vi "DetectionObjectiveStand_Analog.vi"(4 "stand Z vol Backward samp info":cluster{"Fs":dbl, "#s":dbl}={"Fs"=500000.0, "#s"=68421.0}, 6 "stand Z vol Acquisition samp info":cluster{"Fs":dbl, "#s":dbl}={"Fs"=500000.0, "#s"=131579.0}, 7 "Objective scan volt":dbl=5.0, 8 "error in (no error)":errorcluster, 9 "stand Z vol Backward time (s)":dbl=0.13684210526315793, 10 "stand Z vol Acquisition time (s)":dbl=0.2631578947368421, 11 "Steps per volume":dbl=25.0) -> (0 "error out":errorcluster, 3 "DetectionObjectiveStand":waveform(dbl))   [LabVIEW 2018]
panel:
  out "Preview":waveform(dbl)(graph)
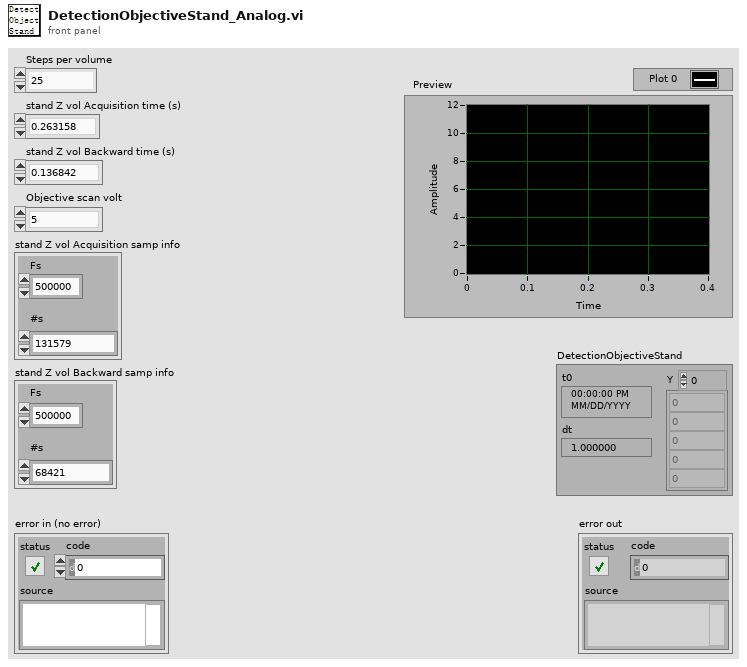
[diagram p1: front panel]
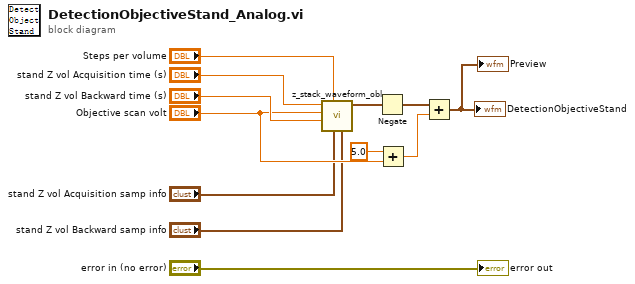
[diagram p0: block diagram]
diagram:
  n1 = call "z_stack_waveform_obl.vi"("Z stack backward"="stand Z vol Backward samp info", "Z stack acquisition"="stand Z vol Acquisition samp info", "Steps per Volume"="Steps per volume", "Backward Time (s)"="stand Z vol Backward time (s)", "SPECIFIC scan volt"="Objective scan volt", "Aquisition Time (s)"="stand Z vol Acquisition time (s)") -> ("WaveformOut"=w9:waveform(dbl))  [unwired: 5 in]
  n2 = Negate(x=w9) -> (-x=w12:waveform(dbl))
  n3 = Add(x=5.0, y="Objective scan volt") -> (x+y=w10:dbl)
  n4 = Add(x=w12, y=w10) -> (x+y=→"DetectionObjectiveStand" →"Preview":waveform(dbl))
  "error out" <- "error in (no error)"
